vi "tkrsa6100 Return String Parser.vi"(0 "Read Buffer":string, 5 "Response String \nFormat(ASCII)":enum16{"ASCII", "BINARY"}(ring), 11 "error in (no error)":errorcluster) -> (4 "Inst Query Response":string, 15 "error out":errorcluster {"code" format="%#.0f"})   [LabVIEW 2020, in "Library Instrument & Equipement.lvlib" / "Library Spectrum Analyser.lvlib"]
doc: "This VI parses the instrument response into the actual instrument response to a query and updates the error out cluster with the currently reported error information.\n\nThe format of the returned string is:\n\n<instrument response string>;<error #>,<\"error information;\">\n\nFirst the entire string is reversed so the quoted error information field at the end can be parsed. This is done with 2 Match Pattern functions that detect the first and second quotes in the reversed string. The resulting string between the quotes is reversed again and used to update the source indicator in error out.\n\nThe rest of the reversed string is passed to tkrsa6100 Error Parser.vi which outputs the actual instrument query response if a query was sent, error #, and error code. The last two complete updating of the error out cluster.\n\nIf the instrument query response is in ASCII format, the response is passed to tkrsa6100 Quote Stripper.vi which removes any quotes from the returned information so that all instrument responses return unquoted information."
uses:
  Library Spectrum Analyser.lvlib
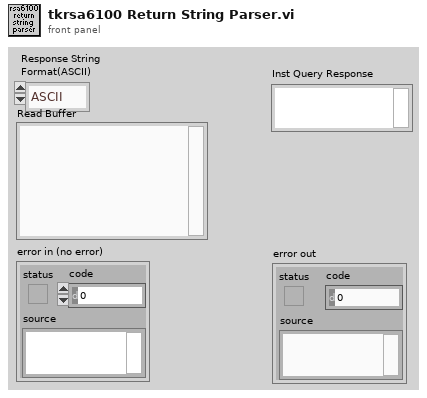
[diagram p1: front panel]
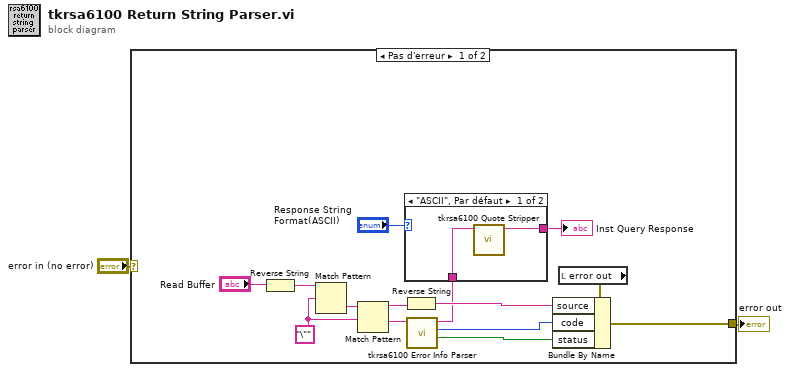
[diagram p0: block diagram]
diagram:
  n1 = case shown="Pas d'erreur" "error in (no error)" {
    selector: "error in (no error)" -> [_ w20]
    tunnel: [w14 w20] -> w2
    frame No Error {
      w12 = "\"" ("regular expression")
      n2 = Reverse String(1:"Read Buffer") -> (0:w3:string)
      n3 = Match Pattern(string=w3, regular expression=w12) -> (after substring=w13:string)  [unwired: 4 out]
      n4 = Match Pattern(string=w13, regular expression=w12) -> (before substring=w11:string, after substring=w9:string)  [unwired: 3 out]
      n5 = Reverse String(1:w11) -> (0:w10:string)
      n6 = call "tkrsa6100 Error Info Parser.vi"("Input String"=w9) -> ("Error Status"=w7:bool, "Error #"=w8:i32, "Response String"=w6:string)  [unwired: 8 out]
      n7 = case shown="\"ASCII\", Par défaut" "Response String \nFormat(ASCII)" {
        tunnel: w6 -> [w18 w19]
        tunnel: [w17 w19] -> w5
        frame "ASCII", Default {
          n8 = call "tkrsa6100 Quote Stripper.vi"("Input String"=w18) -> ("Output String"=w17:string)  [unwired: 10 out]
        }
        frame "BINARY" {
        }
      }
      "Inst Query Response" <- w5
      n9 = local read "error out"() -> (w15:errorcluster)
      n10 = Bundle By Name(cluster=w15, "source"=w10, "code"=w8, "status"=w7) -> (w14:errorcluster)
    }
    frame Error {
      # "if pending error pass it through"
    }
  }
  "error out" <- w2
